vi "Send_String_data.vi"(8 "error in (no error)":errorcluster, 10 "Data":string, 11 "Test_Nested in":refnum<class "Test_Nested.lvclass">) -> (0 "error out":errorcluster, 3 "Test_Nested out":refnum<class "Test_Nested.lvclass">)   [LabVIEW 2025, in "Test_Nested.lvlib" / "Test_Nested.lvclass"]
uses:
  Test_Nested.lvclass
  C:/Program Files (x86)/National Instruments/LabVIEW 2025/vi.lib/ActorFramework/Actor/Actor.lvclass
  <vilib>/ActorFramework/Actor/Actor.lvclass/Actor.ctl
  Test_Nested.lvclass/Test_Nested.ctl
  Test_Nested Messages/New Data Msg/New Data Msg.lvclass/New Data Msg.ctl
  <vilib>/ActorFramework/Message Enqueuer/Message Enqueuer.lvclass/Message Enqueuer.ctl
  <vilib>/ActorFramework/Message Enqueuer/Enqueue.vi
  Test_Nested Messages/New Data Msg/New Data Msg.lvclass
  C:/Program Files (x86)/National Instruments/LabVIEW 2025/vi.lib/ActorFramework/Message/Message.lvclass
  <vilib>/ActorFramework/Message Priority Queue/Priority Enqueue.vi
  <vilib>/ActorFramework/Actor/Actor.lvclass
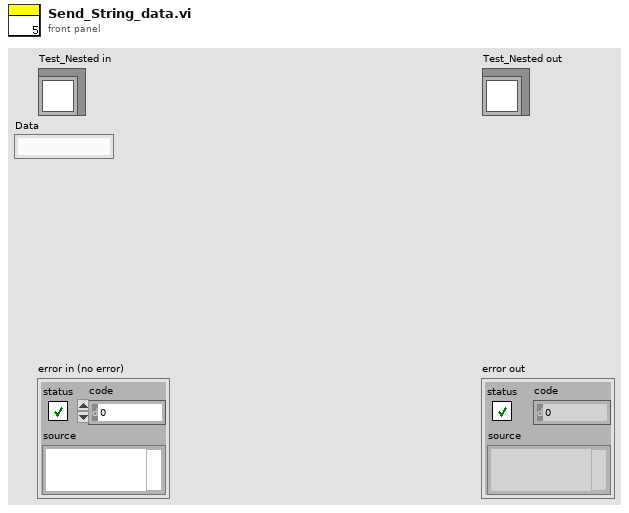
[diagram p1: front panel]
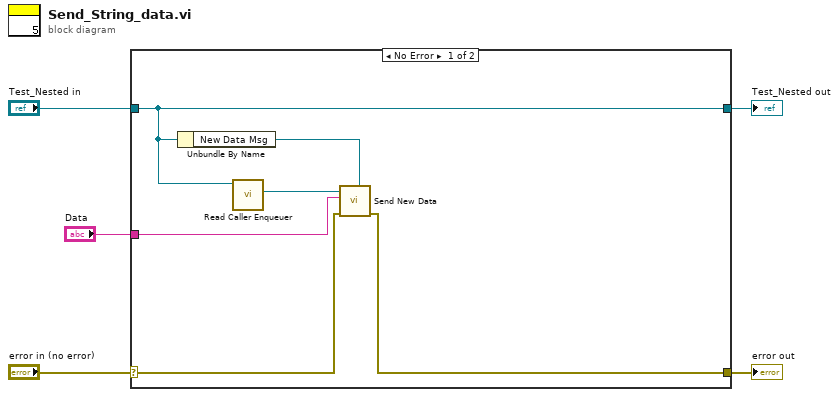
[diagram p0: block diagram]
diagram:
  n1 = case shown="No Error" "error in (no error)" {
    selector: "error in (no error)" -> [w7 w13]
    tunnel: [w6 w13] -> w4
    tunnel: [w10 w12] -> w2
    tunnel: "Test_Nested in" -> [w10 w12]
    tunnel: "Data" -> [w8 _]
    frame No Error {
      n2 = Unbundle By Name(w10) -> ("New Data Msg"=w11:refnum<class "New Data Msg.lvclass">)
      n3 = call <vilib>:"Read Caller Enqueuer.vi"("Actor"=w10) -> ("Caller Enqueuer"=w9:refnum<class "Message Enqueuer.lvclass">)  [unwired: 10 in]
      n4 = call "Send New Data.vi"("Message Type"=w11, "error in (no error)"=w7, "Data"=w8, "Message Enqueuer"=w9) -> ("error out"=w6:errorcluster)  [unwired: 6 in, 1 out]
    }
    frame Error {
    }
  }
  "error out" <- w4
  "Test_Nested out" <- w2
